vi "HyperTerm Data Decode.vi"(0 "Water Heater GEA2 Data in":T1 {"CRC" format="%x"; "Length" format="%x"; "Command" format="%x"; "Destination" format="%x"; "Source" format="%x"}, 1 "Hex Array Out":string[](array[string])) -> (6 "Reason for Data Word 4":string, 7 "Reason for last heating cycle termination":u16, 8 "T2 Tank Sensor":dbl, 9 "EEV Position (0-480)":u16, 10 "T3A (EvapIN)":dbl, 11 "Water Heater GEA2 Data out":T1 {"CRC" format="%x"; "Length" format="%x"; "Command" format="%x"; "Destination" format="%x"; "Source" format="%x"}, 12 "Reason for Data Word 3":string, 13 "Voltage (Volts)":u16, 14 "T3B (EvapOut)":dbl, 15 "Reason for Data Word 2":string, 16 "T4(CompressorDischarge)":dbl, 17 "Reason for Data Word 1":string, 18 "T5(Ambient)":dbl)   [LabVIEW 2014, in "GEA2_Toolkit.lvlib"]
uses:
  Labview GEA2 Toolkit v2.1/library/GEA2_Toolkit.lvlib
  type defs/WaterHeater GEA2 Data.ctl
  type defs/Status Query.ctl
  GEA2 Commands/HEWH/Type Definitions/GEA2 Commands Button Status.ctl
  GEA2 Commands/HEWH/Type Definitions/GEA2 Commands Service Error Codes.ctl
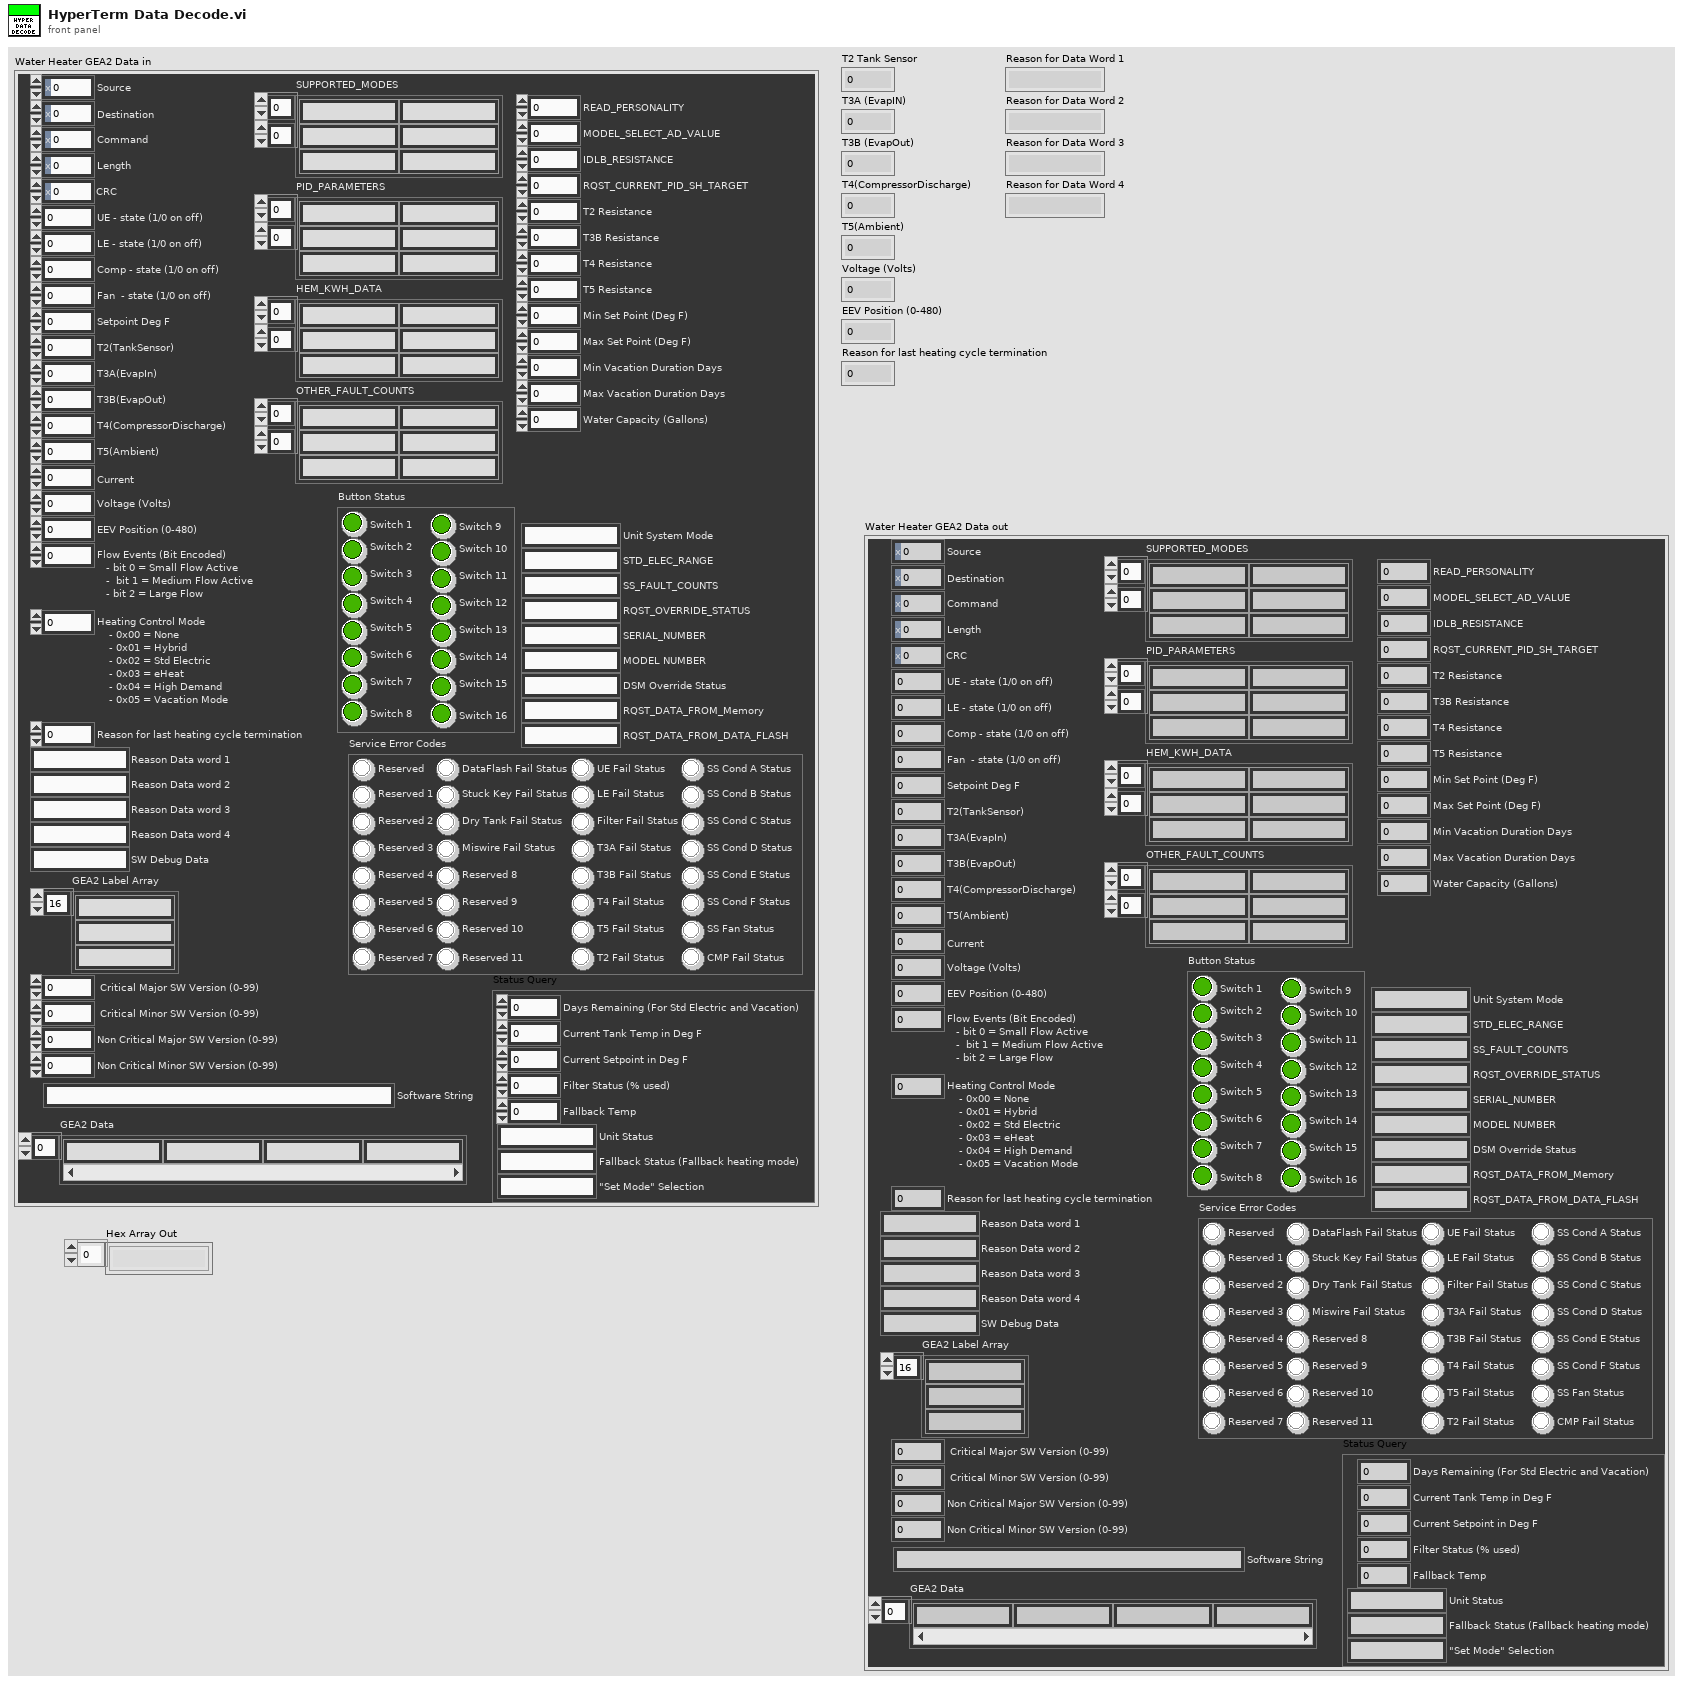
[diagram p1: front panel]
types:
  T1 = typedef "GEA2_Toolkit.lvlib/WaterHeater GEA2 Data.ctl" = cluster{"UE - state (1/0 on off)":u8, "LE - state (1/0 on off)":u8, "Comp - state (1/0 on off)":u8, "Fan  - state (1/0 on off)":u8, "Setpoint Deg F":i32, "T2(TankSensor)":dbl, "T3A(EvapIn)":dbl, "T3B(EvapOut)":dbl, "T4(CompressorDischarge)":dbl, "T5(Ambient)":dbl, "Current":dbl, "Voltage (Volts)":u16, "EEV Position (0-480)":u16, "Flow Events (Bit Encoded)":u16, "Heating Control Mode":u16, "Reason for last heating cycle termination":u16, "Reason Data word 1":string, "Reason Data word 2":string, "Reason Data word 3":string, "Reason Data word 4":string, "SW Debug Data":string, "Source":u8, "Destination":u8, "Command":u8, "Length":u8, "CRC":u16, "GEA2 Label Array":string[], " Critical Major SW Version (0-99)":u16, " Critical Minor SW Version (0-99)":u16, "Non Critical Major SW Version (0-99)":u16, "Non Critical Minor SW Version (0-99)":u16, "Software String":string, "GEA2 Data":string[], "Unit System Mode":string, "RQST_CURRENT_PID_SH_TARGET":u16, "RQST_DATA_FROM_DATA_FLASH":string, "RQST_DATA_FROM_Memory":string, "DSM Override Status":string, "IDLB_RESISTANCE":u32, "MODEL NUMBER":string, "MODEL_SELECT_AD_VALUE":u32, "RQST_OVERRIDE_STATUS":string, "PID_PARAMETERS":string[][], "READ_PERSONALITY":u8, "SERIAL_NUMBER":string, "SS_FAULT_COUNTS":string, "STD_ELEC_RANGE":string, "SUPPORTED_MODES":string[][], "T2 Resistance":u32, "T3B Resistance":u32, "T4 Resistance":u32, "T5 Resistance":u32, "Min Set Point (Deg F)":u32, "Max Set Point (Deg F)":u32, "Min Vacation Duration Days":u32, "Max Vacation Duration Days":u32, "Water Capacity (Gallons)":u32, "Button Status":T2, "Status Query":T3, "Service Error Codes":T4, "HEM_KWH_DATA":string[][], "OTHER_FAULT_COUNTS":string[][]}
  T2 = typedef "GEA2 Commands Button Status.ctl" = cluster{"Switch 1":bool, "Switch 2":bool, "Switch 3":bool, "Switch 4":bool, "Switch 5":bool, "Switch 6":bool, "Switch 7":bool, "Switch 8":bool, "Switch 9":bool, "Switch 10":bool, "Switch 11":bool, "Switch 12":bool, "Switch 13":bool, "Switch 14":bool, "Switch 15":bool, "Switch 16":bool}
  T3 = typedef "GEA2_Toolkit.lvlib/Status Query.ctl" = cluster{"Days Remaining (For Std Electric and Vacation)":u8, "Unit Status":string, "Current Tank Temp in Deg F":u8, "Current Setpoint in Deg F":u8, "Filter Status (% used)":u8, "Fallback Status (Fallback heating mode)":string, "Fallback Temp":u8, "\"Set Mode\" Selection":string}
  T4 = typedef "GEA2 Commands Service Error Codes.ctl" = cluster{"Reserved":bool, "Reserved 1":bool, "Reserved 2":bool, "Reserved 3":bool, "Reserved 4":bool, "Reserved 5":bool, "Reserved 6":bool, "Reserved 7":bool, "DataFlash Fail Status":bool, "Stuck Key Fail Status":bool, "Dry Tank Fail Status":bool, "Miswire Fail Status":bool, "Reserved 8":bool, "Reserved 9":bool, "Reserved 10":bool, "Reserved 11":bool, "UE Fail Status":bool, "LE Fail Status":bool, "Filter Fail Status":bool, "T3A Fail Status":bool, "T3B Fail Status":bool, "T4 Fail Status":bool, "T5 Fail Status":bool, "T2 Fail Status":bool, "SS Cond A Status":bool, "SS Cond B Status":bool, "SS Cond C Status":bool, "SS Cond D Status":bool, "SS Cond E Status":bool, "SS Cond F Status":bool, "SS Fan Status":bool, "CMP Fail Status":bool}
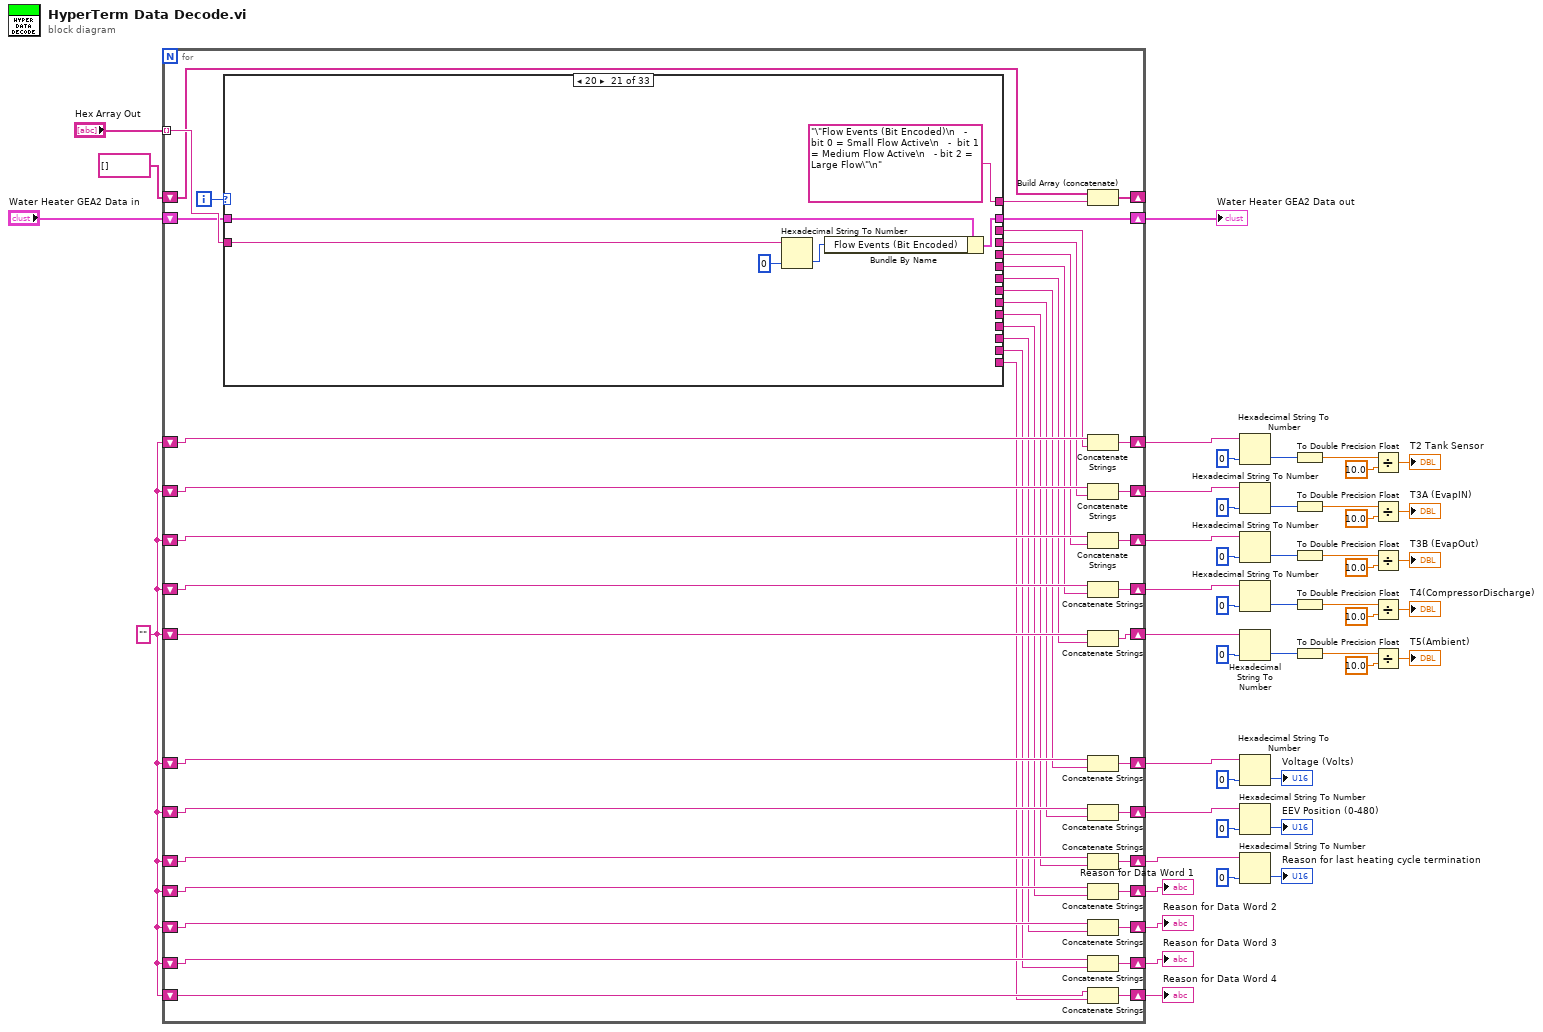
[diagram p0: block diagram]
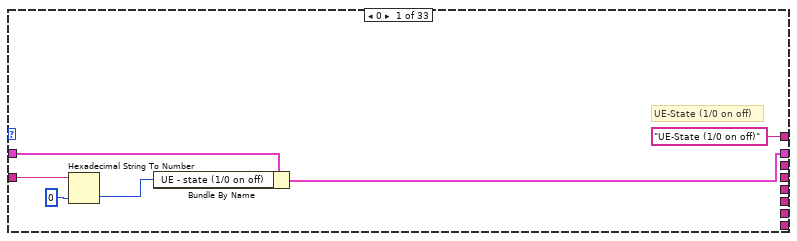
[diagram p2: hidden frame]
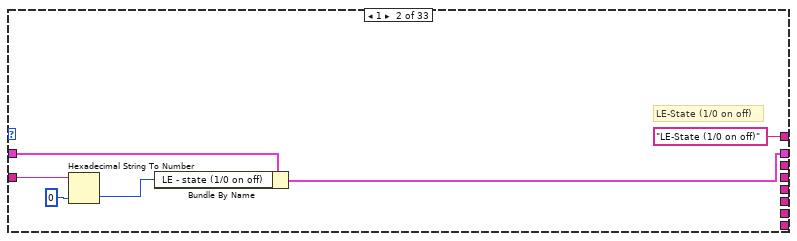
[diagram p3: hidden frame]
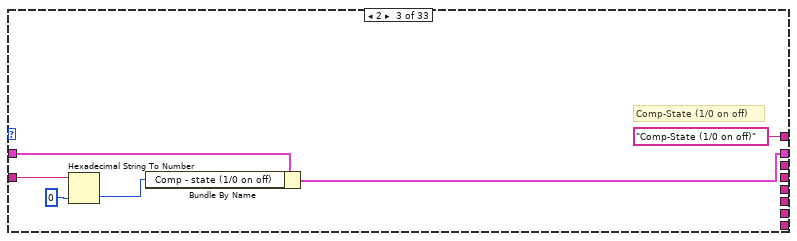
[diagram p4: hidden frame]
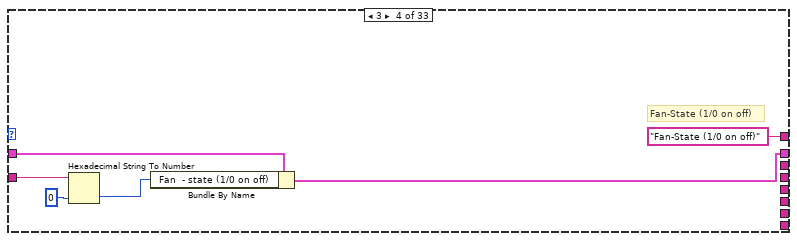
[diagram p5: hidden frame]
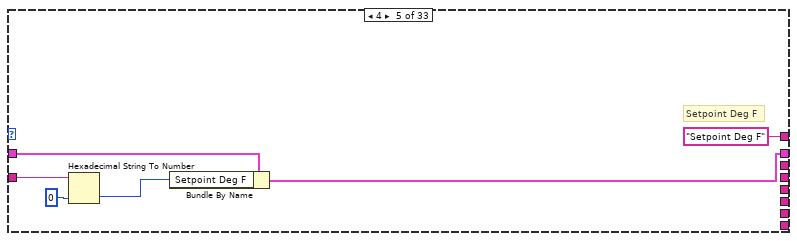
[diagram p6: hidden frame]
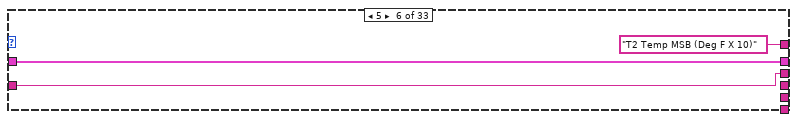
[diagram p7: hidden frame]
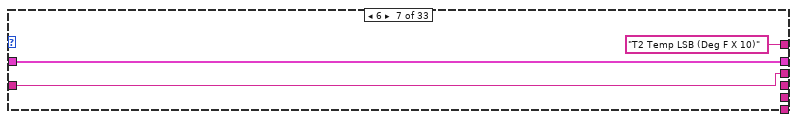
[diagram p8: hidden frame]
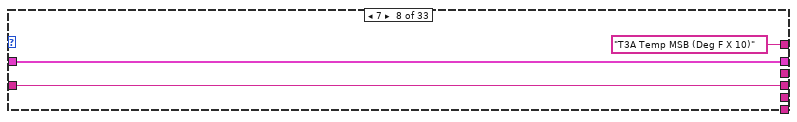
[diagram p9: hidden frame]
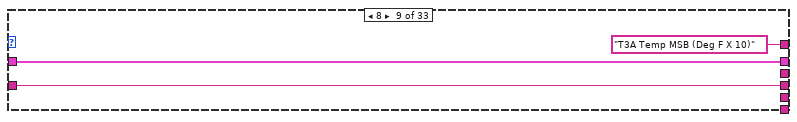
[diagram p10: hidden frame]
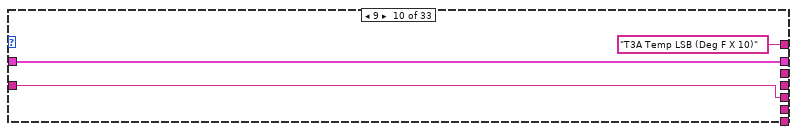
[diagram p11: hidden frame]
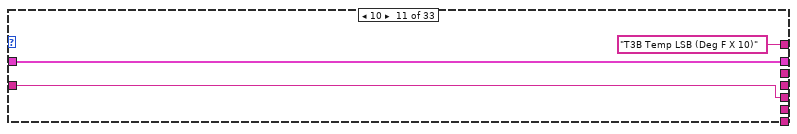
[diagram p12: hidden frame]
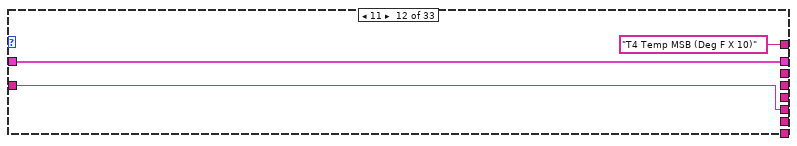
[diagram p13: hidden frame]
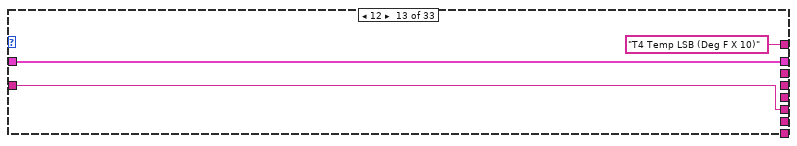
[diagram p14: hidden frame]
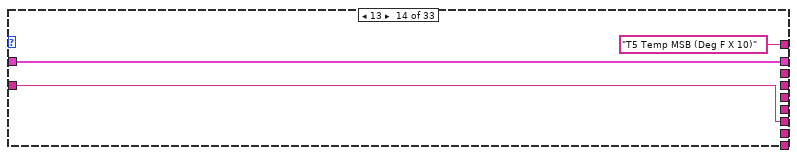
[diagram p15: hidden frame]
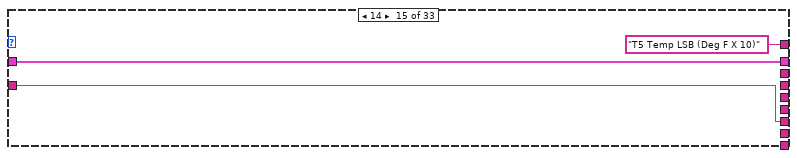
[diagram p16: hidden frame]
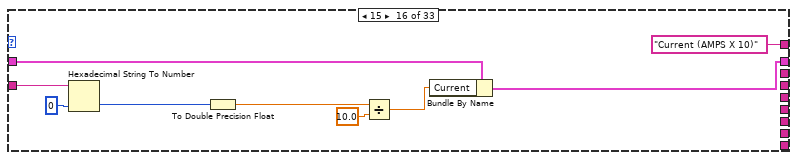
[diagram p17: hidden frame]
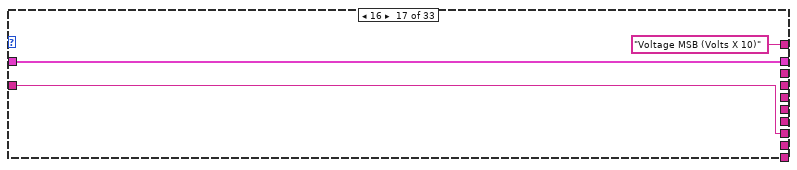
[diagram p18: hidden frame]
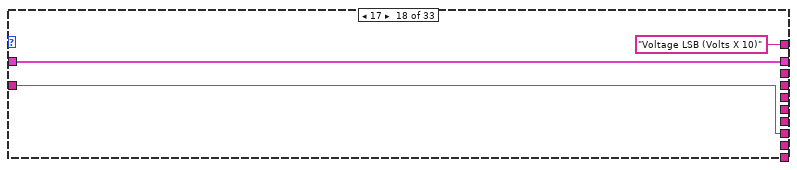
[diagram p19: hidden frame]
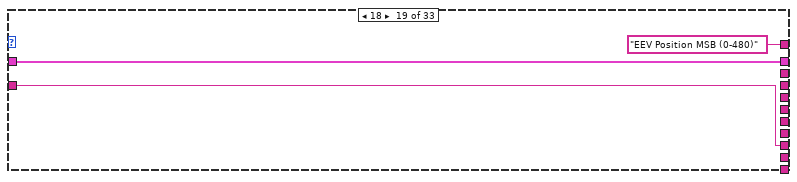
[diagram p20: hidden frame]
diagram:
  w46 = ""
  n1 = for {
    tunnel: "Hex Array Out" -> [w90] mode=indexing
    shift-right: [w87] -> _
    shift-left: string[] [] -> [w89]
    shift-right: [w83] -> w44
    shift-left: "Water Heater GEA2 Data in" -> [w84]
    shift-right: [w50] -> w43
    shift-left: w46 -> [w86]
    shift-right: [w81] -> w42
    shift-left: w46 -> [w82]
    shift-right: [w78] -> w41
    shift-left: w46 -> [w80]
    shift-right: [w75] -> w40
    shift-left: w46 -> [w77]
    shift-right: [w72] -> w39
    shift-left: w46 -> [w74]
    shift-right: [w69] -> w38
    shift-left: w46 -> [w71]
    shift-right: [w66] -> w36
    shift-left: w46 -> [w68]
    shift-right: [w63] -> w34
    shift-left: w46 -> [w65]
    shift-right: [w60] -> w32
    shift-left: w46 -> [w62]
    shift-right: [w57] -> w31
    shift-left: w46 -> [w59]
    shift-right: [w54] -> w30
    shift-left: w46 -> [w56]
    shift-right: [w51] -> w29
    shift-left: w46 -> [w53]
    i -> [w91]
    n2 = case shown="20" w91 {
      tunnel: w90 -> [w94 w98 w104 w110 w116 w122 w125 w129 w132 w135 w138 w141 w144 w147 w150 w156 w162 w165 w168 w171 w176 w182 w186 w189 w192 w195 w198 w201 w204 w207 w210 w213 w216]
      tunnel: ["UE-State (1/0 on off)" "LE-State (1/0 on off)" "Comp-State (1/0 on off)" "Fan-State (1/0 on off)" "Setpoint Deg F" "T2 Temp MSB (Deg F X 10)" "T2 Temp LSB (Deg F X 10)" "T3A Temp MSB (Deg F X 10)" "T3A Temp MSB (Deg F X 10)" "T3A Temp LSB (Deg F X 10)" "T3B Temp LSB (Deg F X 10)" "T4 Temp MSB (Deg F X 10)" "T4 Temp LSB (Deg F X 10)" "T5 Temp MSB (Deg F X 10)" "T5 Temp LSB (Deg F X 10)" "Current (AMPS X 10)" "Voltage MSB (Volts X 10)" "Voltage LSB (Volts X 10)" "EEV Position MSB (0-480)" "EEV Position LSB (0-480)" "\"Flow Events (Bit Encoded)\n   - bit 0 = Small Flow Active\n   -  bit 1 = Medium Flow Active\n   - bit 2 = Large Flow\"\n" "Heating Control Mode\n    - 0x00 = None\n    - 0x01 = Hybrid\n    - 0x02 = Std Electric\n    - 0x03 = eHeat\n    - 0x04 = High Demand\n    - 0x05 = Vacation Mode" "Reason for last heating cycle termination, MSB\n" "Reason for last heating cycle termination, LSB" "Reason Data word 1, MSB" "Reason Data word 1, LSB" "Reason Data word 2, MSB" "Reason Data word 2, LSB" "Reason Data word 3, MSB" "Reason Data word 3, LSB" "Reason Data word 4, MSB" "Reason Data word 4, LSB" "SW Debug Data"] -> w88
      tunnel: [_ _ _ _ _ w122 w125 _ _ _ _ _ _ _ _ _ _ _ _ _ _ _ _ _ _ _ _ _ _ _ _ _ _] -> w85
      tunnel: w84 -> [w96 w101 w107 w113 w117 w123 w126 w128 w131 w134 w137 w140 w143 w146 w149 w159 w161 w164 w167 w170 w175 w181 w185 w188 w191 w194 w197 w200 w203 w206 w209 w212 w218]
      tunnel: [w95 w100 w106 w112 w118 w123 w126 w128 w131 w134 w137 w140 w143 w146 w149 w158 w161 w164 w167 w170 w174 w180 w185 w188 w191 w194 w197 w200 w203 w206 w209 w212 w219] -> w83
      tunnel: [_ _ _ _ _ _ _ w129 w132 _ _ _ _ _ _ _ _ _ _ _ _ _ _ _ _ _ _ _ _ _ _ _ _] -> w49
      tunnel: [_ _ _ _ _ _ _ _ _ w135 w138 _ _ _ _ _ _ _ _ _ _ _ _ _ _ _ _ _ _ _ _ _ _] -> w79
      tunnel: [_ _ _ _ _ _ _ _ _ _ _ w141 w144 _ _ _ _ _ _ _ _ _ _ _ _ _ _ _ _ _ _ _ _] -> w76
      tunnel: [_ _ _ _ _ _ _ _ _ _ _ _ _ w147 w150 _ _ _ _ _ _ _ _ _ _ _ _ _ _ _ _ _ _] -> w73
      tunnel: [_ _ _ _ _ _ _ _ _ _ _ _ _ _ _ _ w162 w165 _ _ _ _ _ _ _ _ _ _ _ _ _ _ _] -> w70
      tunnel: [_ _ _ _ _ _ _ _ _ _ _ _ _ _ _ _ _ _ w168 w171 _ _ _ _ _ _ _ _ _ _ _ _ _] -> w67
      tunnel: [_ _ _ _ _ _ _ _ _ _ _ _ _ _ _ _ _ _ _ _ _ _ w186 w189 _ _ _ _ _ _ _ _ _] -> w64
      tunnel: [_ _ _ _ _ _ _ _ _ _ _ _ _ _ _ _ _ _ _ _ _ _ _ _ w192 w195 _ _ _ _ _ _ _] -> w61
      tunnel: [_ _ _ _ _ _ _ _ _ _ _ _ _ _ _ _ _ _ _ _ _ _ _ _ _ _ w198 w201 _ _ _ _ _] -> w58
      tunnel: [_ _ _ _ _ _ _ _ _ _ _ _ _ _ _ _ _ _ _ _ _ _ _ _ _ _ _ _ w204 w207 _ _ _] -> w55
      tunnel: [_ _ _ _ _ _ _ _ _ _ _ _ _ _ _ _ _ _ _ _ _ _ _ _ _ _ _ _ _ _ w210 w213 _] -> w52
      frame 0 {
        # "UE-State (1/0 on off)"
        n3 = Hexadecimal String To Number(string=w94, default (0uL)=u8 0 ("default (0 U32)")) -> (number=w92:u8)  [unwired: 1 in, 1 out]
        n4 = Bundle By Name(cluster=w96, "UE - state (1/0 on off)"=w92) -> (w95:T1)
      }
      frame 1 {
        # "LE-State (1/0 on off)"
        n5 = Hexadecimal String To Number(string=w98, default (0uL)=u8 0 ("default (0 U32)")) -> (number=w99:u8)  [unwired: 1 in, 1 out]
        n6 = Bundle By Name(cluster=w101, "LE - state (1/0 on off)"=w99) -> (w100:T1)
      }
      frame 2 {
        # "Comp-State (1/0 on off)"
        n7 = Hexadecimal String To Number(string=w104, default (0uL)=u8 0 ("default (0 U32)")) -> (number=w105:u8)  [unwired: 1 in, 1 out]
        n8 = Bundle By Name(cluster=w107, "Comp - state (1/0 on off)"=w105) -> (w106:T1)
      }
      frame 3 {
        # "Fan-State (1/0 on off)"
        n9 = Hexadecimal String To Number(string=w110, default (0uL)=u8 0 ("default (0 U32)")) -> (number=w111:u8)  [unwired: 1 in, 1 out]
        n10 = Bundle By Name(cluster=w113, "Fan  - state (1/0 on off)"=w111) -> (w112:T1)
      }
      frame 4 {
        # "Setpoint Deg F"
        n11 = Hexadecimal String To Number(string=w116, default (0uL)=0 ("default (0 U32)")) -> (number=w119:i32)  [unwired: 1 in, 1 out]
        n12 = Bundle By Name(cluster=w117, "Setpoint Deg F"=w119) -> (w118:T1)
      }
      frame 5 {
      }
      frame 6 {
      }
      frame 7 {
      }
      frame 8 {
      }
      frame 9 {
      }
      frame 10 {
      }
      frame 11 {
      }
      frame 12 {
      }
      frame 13 {
      }
      frame 14 {
      }
      frame 15 {
        n13 = Hexadecimal String To Number(string=w156, default (0uL)=u16 0 ("default (0 U32)")) -> (number=w153:u16)  [unwired: 1 in, 1 out]
        n14 = To Double Precision Float(number=w153) -> (double precision float=w154:dbl)
        n15 = Divide(x=w154, y=10.0) -> (x/y=w152:dbl)
        n16 = Bundle By Name(cluster=w159, "Current"=w152) -> (w158:T1)
      }
      frame 16 {
      }
      frame 17 {
      }
      frame 18 {
      }
      frame 19 {
      }
      frame 20 {
        n17 = Hexadecimal String To Number(string=w176, default (0uL)=u16 0 ("default (0 U32)")) -> (number=w173:u16)  [unwired: 1 in, 1 out]
        n18 = Bundle By Name(cluster=w175, "Flow Events (Bit Encoded)"=w173) -> (w174:T1)
      }
      frame 21 {
        n19 = Hexadecimal String To Number(string=w182, default (0uL)=u16 0 ("default (0 U32)")) -> (number=w179:u16)  [unwired: 1 in, 1 out]
        n20 = Bundle By Name(cluster=w181, "Heating Control Mode"=w179) -> (w180:T1)
      }
      frame 22 {
      }
      frame 23 {
      }
      frame 24 {
      }
      frame 25 {
      }
      frame 26 {
      }
      frame 27 {
      }
      frame 28 {
      }
      frame 29 {
      }
      frame 30 {
      }
      frame 31 {
      }
      frame 32, Default {
        n21 = Unbundle By Name(w218) -> ("SW Debug Data"=w217:string)
        n22 = Concatenate Strings(w217, w216) -> (w215:string)
        n23 = Bundle By Name(cluster=w218, "SW Debug Data"=w215) -> (w219:T1)
      }
    }
    n24 = Build Array (concatenate)(w89, w88) -> (w87:string[])
    n25 = Concatenate Strings(w86, w85) -> (w50:string)
    n26 = Concatenate Strings(w82, w49) -> (w81:string)
    n27 = Concatenate Strings(w80, w79) -> (w78:string)
    n28 = Concatenate Strings(w77, w76) -> (w75:string)
    n29 = Concatenate Strings(w74, w73) -> (w72:string)
    n30 = Concatenate Strings(w71, w70) -> (w69:string)
    n31 = Concatenate Strings(w68, w67) -> (w66:string)
    n32 = Concatenate Strings(w65, w64) -> (w63:string)
    n33 = Concatenate Strings(w62, w61) -> (w60:string)
    n34 = Concatenate Strings(w59, w58) -> (w57:string)
    n35 = Concatenate Strings(w56, w55) -> (w54:string)
    n36 = Concatenate Strings(w53, w52) -> (w51:string)
  }
  "Water Heater GEA2 Data out" <- w44
  "Reason for Data Word 1" <- w32
  "Reason for Data Word 2" <- w31
  "Reason for Data Word 3" <- w30
  "Reason for Data Word 4" <- w29
  n37 = Hexadecimal String To Number(string=w43, default (0uL)=u16 0) -> (number=w19:u16)  [unwired: 1 in, 1 out]
  n38 = Hexadecimal String To Number(string=w42, default (0uL)=u16 0) -> (number=w14:u16)  [unwired: 1 in, 1 out]
  n39 = Hexadecimal String To Number(string=w41, default (0uL)=u16 0) -> (number=w10:u16)  [unwired: 1 in, 1 out]
  n40 = Hexadecimal String To Number(string=w40, default (0uL)=u16 0) -> (number=w6:u16)  [unwired: 1 in, 1 out]
  n41 = Hexadecimal String To Number(string=w39, default (0uL)=u16 0) -> (number=w2:u16)  [unwired: 1 in, 1 out]
  n42 = Hexadecimal String To Number(string=w38, default (0uL)=u16 0) -> (number=→"Voltage (Volts)":u16)  [unwired: 1 in, 1 out]
  n43 = Hexadecimal String To Number(string=w36, default (0uL)=u16 0) -> (number=→"EEV Position (0-480)":u16)  [unwired: 1 in, 1 out]
  n44 = Hexadecimal String To Number(string=w34, default (0uL)=u16 0) -> (number=→"Reason for last heating cycle termination":u16)  [unwired: 1 in, 1 out]
  n45 = To Double Precision Float(number=w19) -> (double precision float=w18:dbl)
  n46 = To Double Precision Float(number=w14) -> (double precision float=w16:dbl)
  n47 = To Double Precision Float(number=w10) -> (double precision float=w11:dbl)
  n48 = To Double Precision Float(number=w6) -> (double precision float=w8:dbl)
  n49 = To Double Precision Float(number=w2) -> (double precision float=w3:dbl)
  n50 = Divide(x=w18, y=10.0) -> (x/y=→"T2 Tank Sensor":dbl)
  n51 = Divide(x=w16, y=10.0) -> (x/y=→"T3A (EvapIN)":dbl)
  n52 = Divide(x=w11, y=10.0) -> (x/y=→"T3B (EvapOut)":dbl)
  n53 = Divide(x=w8, y=10.0) -> (x/y=→"T4(CompressorDischarge)":dbl)
  n54 = Divide(x=w3, y=10.0) -> (x/y=→"T5(Ambient)":dbl)
